vi "Get Direct Sampling.vi"(8 "error in (no error)":errorcluster, 11 "RTL-SDR in":refnum<class "RTL-SDR.lvclass">) -> (0 "error out":errorcluster, 1 "function return":i32, 2 "Direct Sampling State":T1, 3 "RTL-SDR out":refnum<class "RTL-SDR.lvclass">)   [LabVIEW 2015, in "RTL-SDR.lvclass"]
uses:
  RTL-SDR.lvclass
  TypeDef/Direct Sampling States.ctl
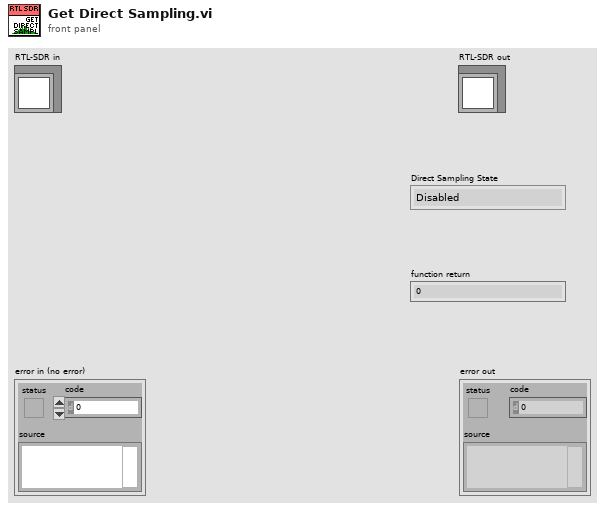
[diagram p1: front panel]
types:
  T1 = typedef "RTL-SDR.lvclass/Direct Sampling States.ctl" = enum16{"Disabled", "I-ADC Input Enabled", "Q-ADC Input Enabled"}
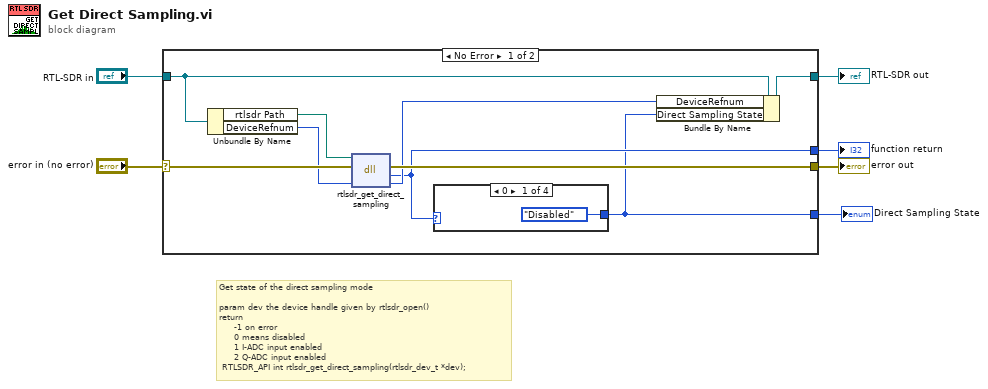
[diagram p0: block diagram]
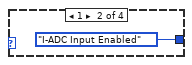
[diagram p2: hidden frame]
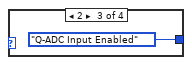
[diagram p3: hidden frame]
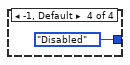
[diagram p4: hidden frame]
diagram:
  # "Get state of the direct sampling mode\n\nparam dev the device handle given by rtlsdr_open()\nreturn \n     -1 on error\n     0 means disabled  \n     1 I-ADC input enabled\n     2 Q-ADC input enabled\n RTLSDR_API int rtlsdr_get_direct_sampling(rtlsdr_dev_t *dev);"
  n1 = case shown="No Error" "error in (no error)" {
    selector: "error in (no error)" -> [w15 w21]
    tunnel: [w14 w21] -> w5
    tunnel: [w10 w20] -> w3
    tunnel: "RTL-SDR in" -> [w13 w20]
    tunnel: [w8 _] -> w2
    tunnel: [w7 _] -> w1
    frame No Error {
      n2 = Unbundle By Name(w13) -> ("rtlsdr Path"=w12:path, "DeviceRefnum"=w11:u64)
      n3 = dll-call lib="C:/Users/Ivan/Desktop/D-23-09-24 (RTL-SDR)/Project (Pelleng-SDR)/rtlsdr/dll/rtlsdr.*" fn="rtlsdr_get_direct_sampling"(path in=w12, error in=w15, "DeviceRefnum"=w11) -> (error out=w14:errorcluster, "return type"=w8:i32, "DeviceRefnum"=w9:u64)  [unwired: 1 in, 1 out]
      n4 = case shown="0" w8 {
        tunnel: [Direct_Sampling_States."Disabled" Direct_Sampling_States."I-ADC Input Enabled" Direct_Sampling_States."Q-ADC Input Enabled" Direct_Sampling_States."Disabled"] -> w7
        frame 0 {
        }
        frame 1 {
        }
        frame 2 {
        }
        frame -1, Default {
        }
      }
      n5 = Bundle By Name(cluster=w13, "DeviceRefnum"=w9, "Direct Sampling State"=w7) -> (w10:refnum<class "RTL-SDR.lvclass">)
    }
    frame Error {
    }
  }
  "error out" <- w5
  "RTL-SDR out" <- w3
  "Direct Sampling State" <- w1
  "function return" <- w2
